vi "Find Element Position.vi"(0 "CtlRef":refnum<vi>, 5 "Coords":T1, 11 "error in (no error)":errorcluster) -> (4 "Row":i32, 6 "Column":i32, 15 "error out":errorcluster)   [LabVIEW 2023, in "Rooms Manager UI.lvlib" / "Rooms Manager UI.lvclass"]
uses:
  Rooms Manager UI.lvclass
  <vilib>/Utility/miscctls.llb/LVPoint32TypeDef.ctl
  Rooms Manager UI.lvclass/Rooms Manager UI.ctl
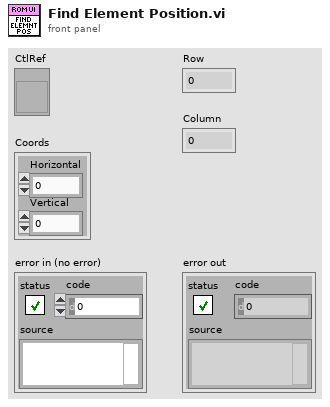
[diagram p1: front panel]
types:
  T1 = typedef "LVPoint32TypeDef.ctl" = cluster{"Horizontal":i32, "Vertical":i32}
  T2 = typedef "LVBoundsTypeDef.ctl" = cluster{"Width":u32, "Height":u32}
  T3 = typedef "LVPositionTypeDef.ctl" = cluster{"Left":i32, "Top":i32}
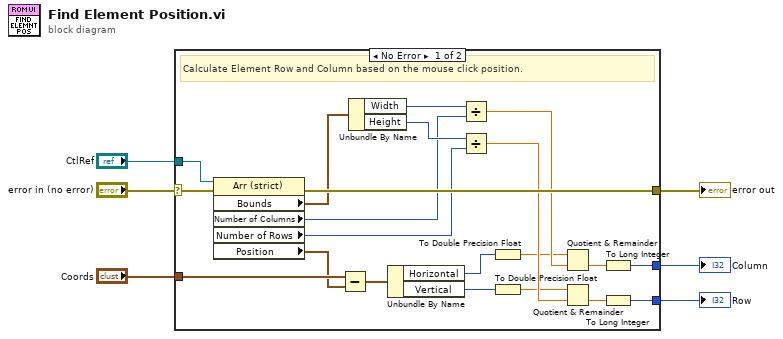
[diagram p0: block diagram]
diagram:
  n1 = case shown="No Error" "error in (no error)" {
    selector: "error in (no error)" -> [w27 w28]
    tunnel: [w26 w28] -> w5
    tunnel: "CtlRef" -> [w25 _]
    tunnel: "Coords" -> [w19 _]
    tunnel: [w9 _] -> w2
    tunnel: [w10 _] -> w1
    frame No Error {
      # "Calculate Element Row and Column based on the mouse click position."
      n2 = property class="Arr (strict)"(reference=w25, error in=w27) -> (error out=w26:errorcluster, "Bounds"=w24:T2, "Number of Columns"=w21:u32, "Number of Rows"=w20:u32, "Position"=w18:T3)  [unwired: 1 out]
      n3 = Subtract(x=w19, y=w18) -> (x-y=w17:T1)
      n4 = Unbundle By Name(w24) -> ("Width"=w23:u32, "Height"=w22:u32)
      n5 = Unbundle By Name(w17) -> ("Horizontal"=w16:i32, "Vertical"=w14:i32)
      n6 = Divide(x=w23, y=w21) -> (x/y=w15:dbl)
      n7 = Divide(x=w22, y=w20) -> (x/y=w13:dbl)
      n8 = To Double Precision Float(number=w16) -> (double precision float=w8:dbl)
      n9 = To Double Precision Float(number=w14) -> (double precision float=w7:dbl)
      n10 = Quotient & Remainder(x=w8, y=w15) -> (floor(x/y)=w11:dbl)  [unwired: 1 out]
      n11 = Quotient & Remainder(x=w7, y=w13) -> (floor(x/y)=w12:dbl)  [unwired: 1 out]
      n12 = To Long Integer(number=w11) -> (32bit integer=w10:i32)
      n13 = To Long Integer(number=w12) -> (32bit integer=w9:i32)
    }
    frame Error {
    }
  }
  "error out" <- w5
  "Column" <- w1
  "Row" <- w2
